vi "getIndex.vi"(8 "error in (no error)":errorcluster, 10 "Active Cell:Cell Background Color":u32(colorbox)=16775911, 11 "TableRef":refnum<vi>) -> (0 "error out":errorcluster)   [LabVIEW 2016, in "ZebraTable.lvlib" / "XControl 1.xctl"]
uses:
  XControl 1.xctl
  <vilib>/Utility/miscctls.llb/LVRowAndColumnUnsignedTypeDef.ctl
panel:
  out "BG Colums":u32[](array[numeric])
  out "BG ROW":u32[](array[numeric])
  out "ALL vi":string[][](table)
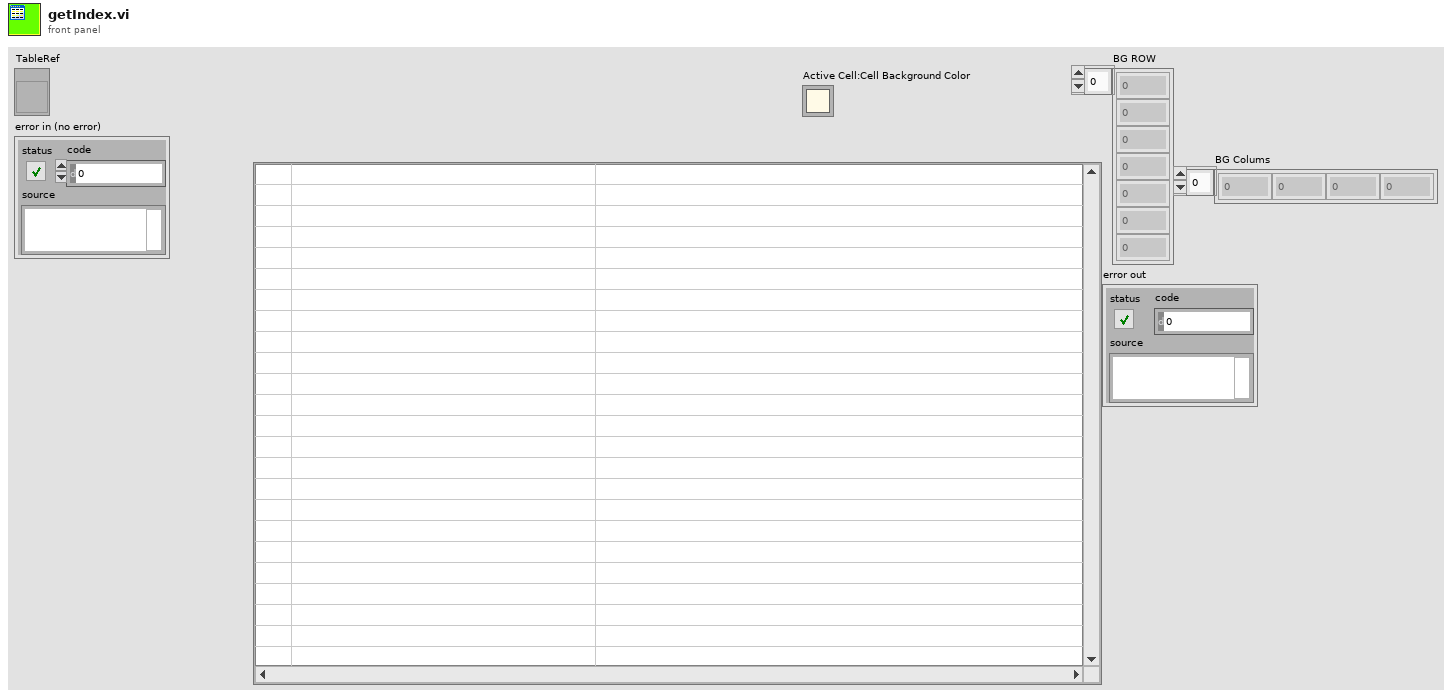
[diagram p1: front panel]
types:
  T1 = typedef "LVRowAndColumnUnsignedTypeDef.ctl" = cluster{"Row":u32, "Column":u32}
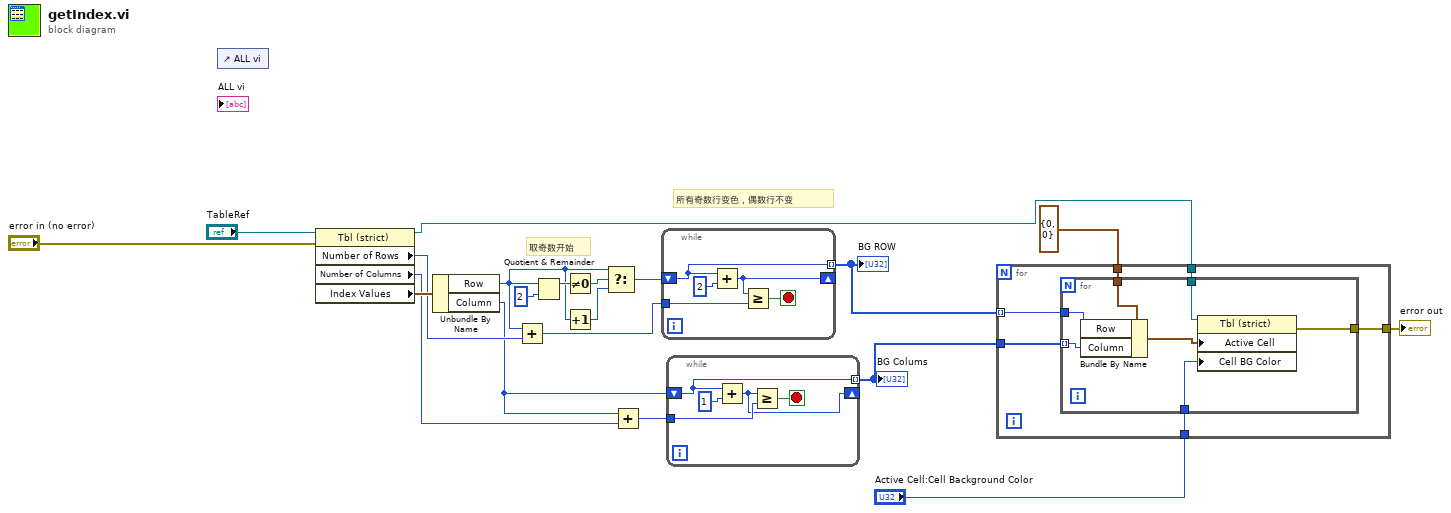
[diagram p0: block diagram]
diagram:
  # "所有奇数行变色，偶数行不变"
  # "取奇数开始"
  n1 = control-ref of="ALL vi"() -> ()  [unwired: 1 out]
  n2 = property class="Tbl (strict)"(reference="TableRef", error in="error in (no error)") -> (reference out=w5:refnum<vi>, "Number of Rows"=w19:u32, "Number of Columns"=w11:u32, "Index Values"=w20:T1)  [unwired: 1 out]
  n3 = Unbundle By Name(w20) -> ("Row"=w12:u32, "Column"=w9:u32)
  n4 = Add(x=w12, y=w19) -> (x+y=w18:u32)
  n5 = Quotient & Remainder(x=w12, y=u32 2) -> (x-y*floor(x/y)=w16:u32)  [unwired: 1 out]
  n6 = Not Equal To 0?(x=w16) -> (x != 0?=w15:bool)
  n7 = Increment(x=w12) -> (x+1=w14:u32)
  n8 = Select(t=w12, s=w15, f=w14) -> (s? t:f=w13:u32)
  n9 = Add(x=w9, y=w11) -> (x+y=w10:u32)
  n10 = while {
    shift-right: [w21] -> _
    shift-left: w13 -> [w24]
    tunnel: [w24] -> w8 mode=indexing
    tunnel: w18 -> [w23]
    stop <- w22 stop-if-true
    n11 = Add(x=w24, y=u32 2) -> (x+y=w21:u32)
    n12 = Greater Or Equal?(x=w21, y=w23) -> (x >= y?=w22:bool)
  }
  "BG ROW" <- w8
  n13 = while {
    shift-right: [w26] -> _
    shift-left: w9 -> [w29]
    tunnel: [w29] -> w7 mode=indexing
    tunnel: w10 -> [w28]
    stop <- w27 stop-if-true
    n14 = Add(x=w29, y=u32 1) -> (x+y=w26:u32)
    n15 = Greater Or Equal?(x=w26, y=w28) -> (x >= y?=w27:bool)
  }
  "BG Colums" <- w7
  n16 = for {
    tunnel: w8 -> [w34] mode=indexing
    tunnel: w7 -> [w36]
    tunnel: T1 {"Row"=0, "Column"=0} ("Index Values") -> [w35]
    tunnel: w5 -> [w33]
    tunnel: "Active Cell:Cell Background Color" -> [w32]
    tunnel: [w31] -> w1
    n17 = for {
      tunnel: w36 -> [w41] mode=indexing
      tunnel: w35 -> [w43]
      tunnel: w34 -> [w42]
      tunnel: w33 -> [w40]
      tunnel: w32 -> [w38]
      tunnel: [w37] -> w31
      n18 = Bundle By Name(cluster=w43, "Row"=w42, "Column"=w41) -> (w39:T1)
      n19 = property class="Tbl (strict)"(reference=w40, "Active Cell"=w39, "Cell BG Color"=w38) -> (error out=w37:errorcluster)  [unwired: 1 in, 1 out]
    }
  }
  "error out" <- w1
